vi "manage.vi"() -> ()   [LabVIEW 2018, in "stepper.lvclass"]
uses:
  stepper.lvclass
  stepper action.ctl
  stack action -- control.ctl
panel:
  in  "stepper action":T1
  in  "stepper IN":refnum<class "stepper.lvclass">
  out "stepper OUT":refnum<class "stepper.lvclass">
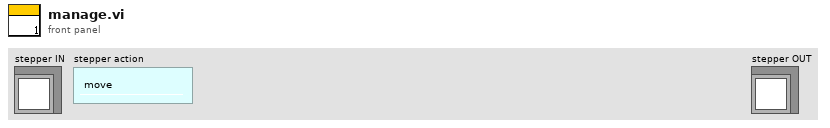
[diagram p1: front panel]
types:
  T1 = typedef "stepper action.ctl" = enum16{"move", "stop", "check", "set", "sync", "void"}
  T2 = typedef "stack action -- control.ctl" = enum16{"push", "pop", "check", "init"}
  T3 = typedef "cursor action.ctl" = enum16{"range", "read", "write", "check", "zoom out", "smart zoom out", "zoom to aspect ratio 1", "zoom to win", "zoom out 20%", "zoom in 20%", "-empty", "smart zoom out&aspect", "move range left 20%", "move range right 20%", "move range up 20%", "move range down 20%", "zoom to X win", "zoom to Y win", "zoom out X", "zoom out Y", "zoom in X", "zoom in Y", "check plot scale"}
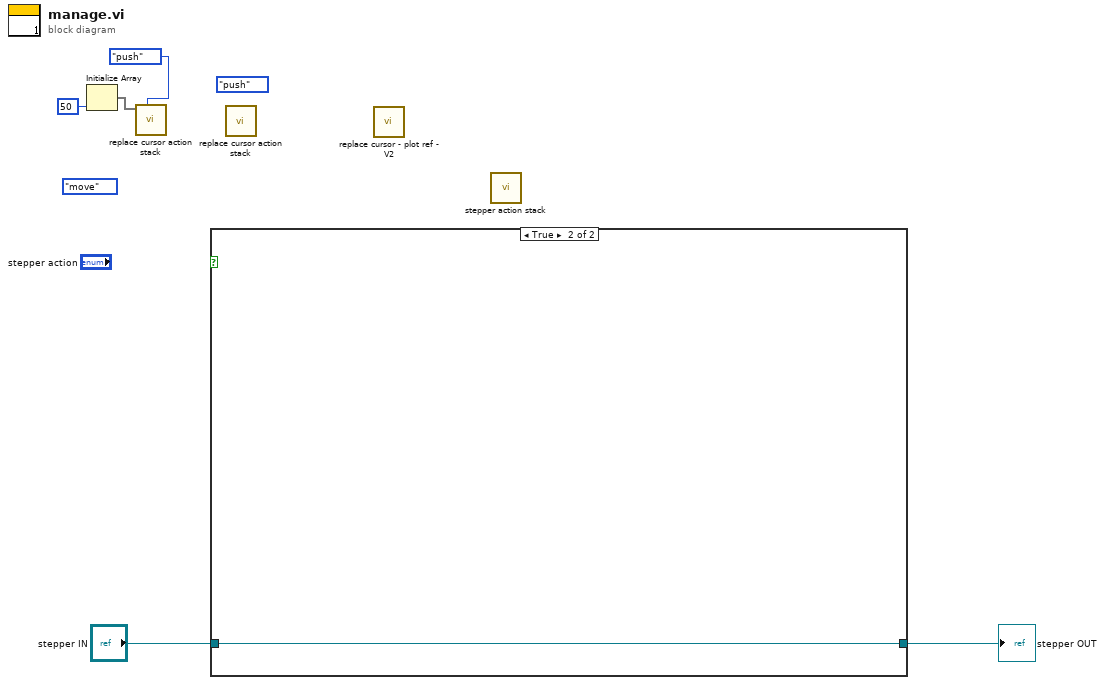
[diagram p0: block diagram]
diagram:
  (unwired) stack_action_--_control."push" ("stack action")
  (unwired) stepper_action."move" ("stepper action")
  n1 = Initialize Array(50 ("dimension size")) -> (w3:T3, w4:void[])
  n2 = call "replace cursor action stack.vi"("stack action"=stack_action_--_control."push", "command stack In"=w4) -> ("command stack Out"=w1:T3[], "cursor action"=w5:T3)  [unwired: 6 in, 2 out]
  n3 = case shown="True" {
    selector: _ -> [_ _]
    tunnel: [_ w9] -> w8
    tunnel: "stepper IN" -> [_ w9]
    frame False {
    }
    frame True {
    }
  }
  "stepper OUT" <- w8
  n4 = call "replace cursor action stack.vi"() -> ()  [unwired: 9 in, 3 out]
  n5 = call "replace cursor - plot ref - V2.vi"() -> ()  [unwired: 16 in, 4 out]
  n6 = call "stepper action stack.vi"() -> ()  [unwired: 10 in, 2 out]
